vi "Test_HW_Stream_raw_data_channel.vi"(7 "At least bits":u32=30, 8 "error in":errorcluster, 9 "Event Type":T1=1073684533 items=["Service Request"=1073684491, "Trigger"=3221168138, "Clear"=1073684493, "VXI Signal"=1073684512, "VXI/VME Interrupt"=3221168161, "VXI/VME Sysfail"=1073684509, "VXI/VME Sysreset"=1073684510, "GPIB CIC"=1073684498, "GPIB Talk"=1073684499, "GPIB Listen"=1073684500, "PXI Interrupt"=1073684514, "Serial Break"=1073684515, "Serial TermChar"=1073684516, "Serial CTS"=1073684521, "Serial DSR"=1073684522, "Serial DCD"=1073684524, "Serial RI"=1073684526, "Serial Character"=1073684533, "USB Interrupt"=1073684535, "All Enabled"=1073709055], 10 "Data flow controls in":T3, 11 "VISA resource name in":refnum<visa-resource-name>) -> (0 "error out":errorcluster, 1 "High-speed channel":T2, 2 "Data flow controls out":T3, 3 "VISA resource name out":refnum<visa-resource-name>, 4 "Timestamp":timestamp, 6 "Time to process, us":dbl format="%0.2f")   [LabVIEW 2018]
uses:
  <extravilib>/ChannelInstances/High Speed Stream-c(a[.](u16),stamp,str)/)Channel.ctl
  <vilib>/Instr/_visa.llb/Select Event Type.ctl
  <vilib>/Instr/_visa.llb/VISA Flush IO Buffer Mask.ctl
  <extravilib>/ChannelInstances/High Speed Stream-c(a[.](u16),stamp,str).lvlib
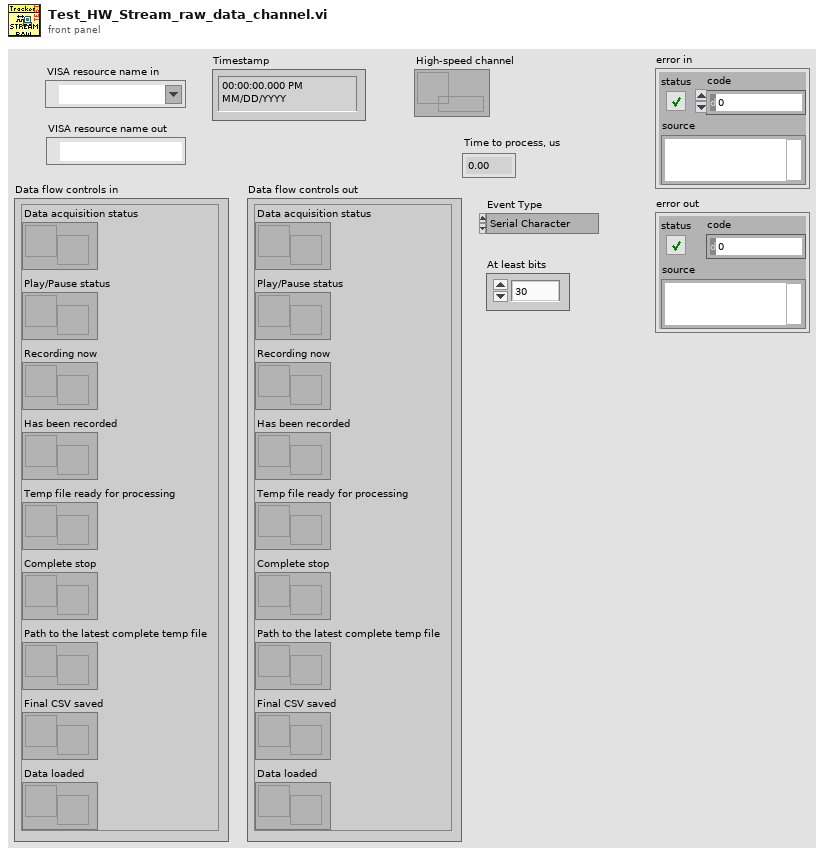
[diagram p1: front panel]
types:
  T1 = typedef "Select Event Type.ctl" = u32
  T2 = typedef "High Speed Stream-c(a[.](u16),stamp,str).lvlib/)Channel.ctl" = refnum<queue>
  T3 = cluster{"Data acquisition status":refnum<notifier>, "Play/Pause status":refnum<notifier>, "Complete stop":refnum<notifier>, "Temp file ready for processing":refnum<notifier>, "Has been recorded":refnum<notifier>, "Recording now":refnum<notifier>, "Path to the latest complete temp file":refnum<notifier>, "Final CSV saved":refnum<notifier>, "Data loaded":refnum<notifier>}
  T4 = typedef "VISA Flush IO Buffer Mask.ctl" = u16
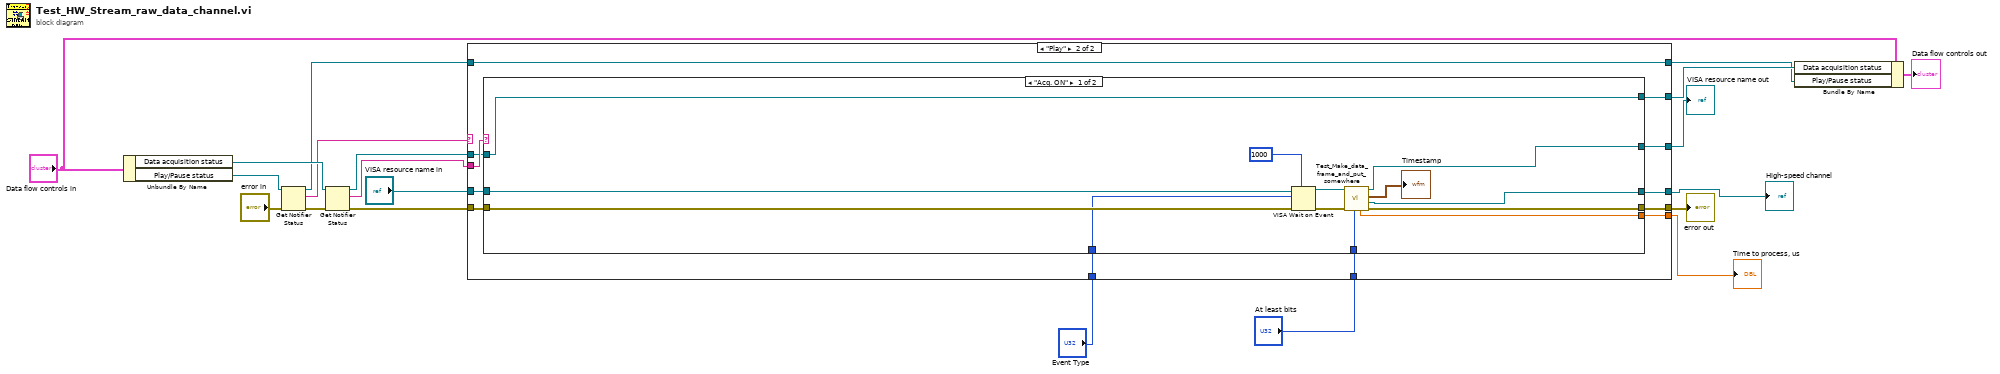
[diagram p0: block diagram]
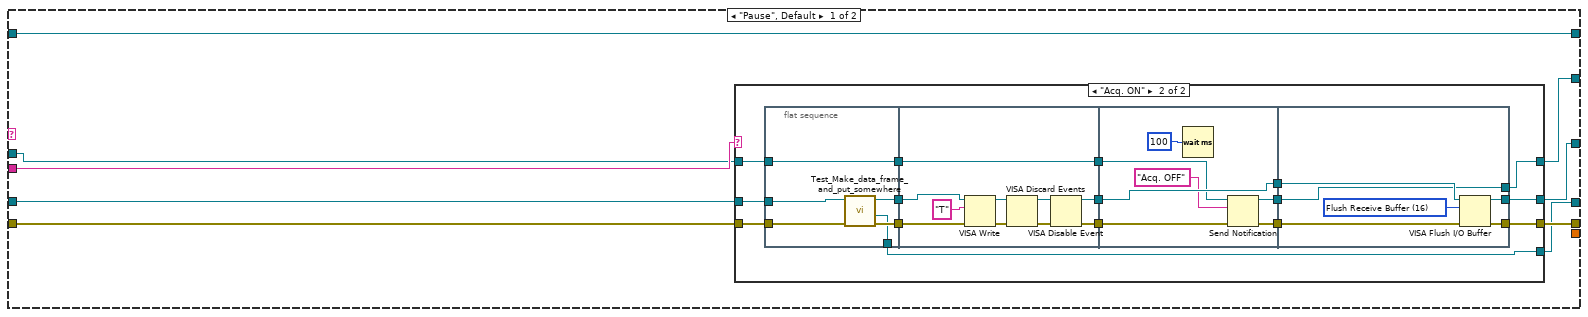
[diagram p2: hidden frame]
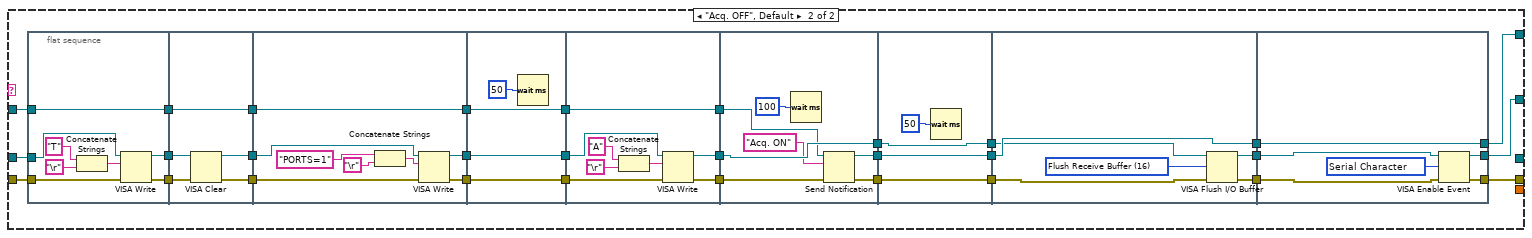
[diagram p4: hidden frame]
diagram:
  n1 = Unbundle By Name("Data flow controls in") -> ("Data acquisition status"=w18:refnum<notifier>, "Play/Pause status"=w17:refnum<notifier>)
  n2 = Get Notifier Status(notifier=w17, error in (no error)="error in") -> (notifier out=w12:refnum<notifier>, current notification=w16:string, error out=w13:errorcluster)  [unwired: 2 out]
  n3 = Get Notifier Status(notifier=w18, error in (no error)=w13) -> (notifier out=w11:refnum<notifier>, current notification=w15:string, error out=w6:errorcluster)  [unwired: 2 out]
  n4 = case shown="\"Play\"" w16 {
    tunnel: [w24 w84] -> w19
    tunnel: "VISA resource name in" -> [w29 w89]
    tunnel: w15 -> [w28 w87]
    tunnel: w12 -> [w26 w85]
    tunnel: w11 -> [w27 w86]
    tunnel: [w23 w83] -> w9
    tunnel: [w26 w85] -> w8
    tunnel: w6 -> [w25 w88]
    tunnel: [w22 w82] -> w5
    tunnel: [_ w81] -> w4
    tunnel: [w21 w80] -> w1
    tunnel: "Event Type" -> [_ w79]
    tunnel: "At least bits" -> [_ w78]
    frame "Pause", Default {
      n5 = case shown="\"Acq. ON\"" w28 {
        tunnel: w29 -> [w32 w46]
        tunnel: [w32 w45] -> w24
        tunnel: w27 -> [w31 w39]
        tunnel: [w31 w38] -> w23
        tunnel: w25 -> [w30 w42]
        tunnel: [w30 w41] -> w22
        tunnel: [_ w33] -> w21
        frame "Acq. OFF", Default {
        }
        frame "Acq. ON" {
          n6 = flat-sequence {
            tunnel: w39 -> [w54]
            tunnel: w42 -> [w53]
            tunnel: w46 -> [w51]
            tunnel: [w50] -> w36
            tunnel: [w52] -> w35
            tunnel: [w54] -> w34
            tunnel: [w49] -> w33
            tunnel: [w56] -> w48
            tunnel: [w55] -> w47
            tunnel: [w64] -> w40
            tunnel: w36 -> [w62]
            tunnel: w35 -> [w61]
            tunnel: w34 -> [w64]
            tunnel: w48 -> [w70]
            tunnel: w47 -> [w69]
            tunnel: [w70] -> w44
            tunnel: [w68] -> w43
            tunnel: w40 -> [w66]
            tunnel: [w65] -> w37
            tunnel: [w75] -> w45
            tunnel: w44 -> [w76]
            tunnel: w43 -> [w77]
            tunnel: [w73] -> w41
            tunnel: [w72] -> w38
            tunnel: w37 -> [w72]
            frame #0 {
              n7 = call "Test_Make_data_frame_and_put_somewhere.vi"("error in"=w53, "VISA resource name in"=w51) -> ("error out"=w52:errorcluster, "High-speed channel"=w49:T2, "VISA resource name out"=w50:refnum<visa-resource-name>)  [unwired: 5 in, 2 out]
            }
            frame #1 {
              n8 = VISA Write(VISA resource name=w62, write buffer="T", error in (no error)=w61) -> (VISA resource name out=w59:refnum<visa-resource-name>, error out=w60:errorcluster)  [unwired: 1 out]
              n9 = VISA Discard Events(8:w60, 11:w59) -> (0:w58:errorcluster, 3:w57:refnum<visa-resource-name>)  [unwired: 2 in]
              n10 = VISA Disable Event(8:w58, 11:w57) -> (0:w55:errorcluster, 3:w56:refnum<visa-resource-name>)  [unwired: 2 in]
            }
            frame #2 {
              n11 = Wait (ms)(milliseconds to wait=u32 100) -> ()  [unwired: 1 out]
              n12 = Send Notification(notification="Acq. OFF", notifier=w66, error in (no error)=w69) -> (notifier out=w65:refnum<notifier>, error out=w68:errorcluster)
            }
            frame #3 {
              w74 = T4 16 items=["Flush Receive Buffer"=16, "Write Transmit Buffer to Device"=32, "Flush Receive Buffer (No I/O)"=64, "Flush Transmit Buffer"=128] ("Mask")
              n13 = VISA Flush I/O Buffer(VISA resource name=w76, mask (16)=w74, error in (no error)=w77) -> (VISA resource name out=w75:refnum<visa-resource-name>, error out=w73:errorcluster)
            }
          }
        }
      }
    }
    frame "Play" {
      n14 = case shown="\"Acq. ON\"" w87 {
        tunnel: w89 -> [w96 w130]
        tunnel: [w99 w103] -> w84
        tunnel: [w100 w104] -> w82
        tunnel: w88 -> [w98 w123]
        tunnel: w86 -> [w102 w118]
        tunnel: [w102 w117] -> w83
        tunnel: [w93 _] -> w81
        tunnel: [w92 _] -> w80
        tunnel: w79 -> [w91 _]
        tunnel: w78 -> [w90 _]
        frame "Acq. ON" {
          n15 = VISA Wait on Event(7:u32 1000 ("timeout (0)"), 8:w98, 10:w91, 11:w96) -> (0:w97:errorcluster, 3:w95:refnum<visa-resource-name>)  [unwired: 1 in, 2 out]
          n16 = call "Test_Make_data_frame_and_put_somewhere.vi"("At least bits"=w90, "error in"=w97, "VISA resource name in"=w95) -> ("error out"=w100:errorcluster, "High-speed channel"=w92:T2, "Timestamp"=→"Timestamp":timestamp, "VISA resource name out"=w99:refnum<visa-resource-name>, "Time to process, us"=w93:dbl)  [unwired: 4 in]
        }
        frame "Acq. OFF", Default {
          n17 = flat-sequence {
            tunnel: w130 -> [w139]
            tunnel: [w140] -> w129
            tunnel: [w138] -> w128
            tunnel: w123 -> [w134]
            tunnel: [w133] -> w119
            tunnel: w118 -> [w133]
            tunnel: [w145] -> w125
            tunnel: [w144] -> w124
            tunnel: w128 -> [w143]
            tunnel: w129 -> [w142]
            tunnel: [w141] -> w120
            tunnel: w119 -> [w141]
            tunnel: w125 -> [w151]
            tunnel: [w150] -> w127
            tunnel: w124 -> [w149]
            tunnel: [w148] -> w126
            tunnel: [w146] -> w121
            tunnel: w120 -> [w146]
            tunnel: [w156] -> w110
            tunnel: [w155] -> w109
            tunnel: [w157] -> w108
            tunnel: w121 -> [w157]
            tunnel: w127 -> [w156]
            tunnel: w126 -> [w155]
            tunnel: [w160] -> w132
            tunnel: [w159] -> w131
            tunnel: w110 -> [w162]
            tunnel: w109 -> [w161]
            tunnel: [w158] -> w122
            tunnel: w108 -> [w158]
            tunnel: w132 -> [w170]
            tunnel: w131 -> [w171]
            tunnel: w122 -> [w168]
            tunnel: [w169] -> w116
            tunnel: [w171] -> w115
            tunnel: [w167] -> w114
            tunnel: w116 -> [w176]
            tunnel: [w176] -> w113
            tunnel: w115 -> [w175]
            tunnel: [w175] -> w112
            tunnel: w114 -> [w174]
            tunnel: [w174] -> w111
            tunnel: w111 -> [w178]
            tunnel: w112 -> [w177]
            tunnel: w113 -> [w179]
            tunnel: [w181] -> w107
            tunnel: [w182] -> w106
            tunnel: [w178] -> w105
            tunnel: [w188] -> w117
            tunnel: w107 -> [w186]
            tunnel: w106 -> [w185]
            tunnel: w105 -> [w188]
            tunnel: [w187] -> w104
            tunnel: [w184] -> w103
            frame #0 {
              n18 = Concatenate Strings("T" ("write buffer"), "\r") -> (w135:string)
              n19 = VISA Write(VISA resource name=w139, write buffer=w135, error in (no error)=w134) -> (VISA resource name out=w140:refnum<visa-resource-name>, error out=w138:errorcluster)  [unwired: 1 out]
            }
            frame #1 {
              n20 = VISA Clear(VISA resource name=w142, error in (no error)=w143) -> (VISA resource name out=w145:refnum<visa-resource-name>, error out=w144:errorcluster)
            }
            frame #2 {
              n21 = Concatenate Strings("PORTS=1" ("write buffer"), "\r") -> (w152:string)
              n22 = VISA Write(VISA resource name=w151, write buffer=w152, error in (no error)=w149) -> (VISA resource name out=w150:refnum<visa-resource-name>, error out=w148:errorcluster)  [unwired: 1 out]
            }
            frame #3 {
              n23 = Wait (ms)(milliseconds to wait=u32 50) -> ()  [unwired: 1 out]
            }
            frame #4 {
              n24 = Concatenate Strings("A" ("write buffer"), "\r") -> (w163:string)
              n25 = VISA Write(VISA resource name=w162, write buffer=w163, error in (no error)=w161) -> (VISA resource name out=w159:refnum<visa-resource-name>, error out=w160:errorcluster)  [unwired: 1 out]
            }
            frame #5 {
              n26 = Wait (ms)(milliseconds to wait=u32 100) -> ()  [unwired: 1 out]
              n27 = Send Notification(notification="Acq. ON", notifier=w168, error in (no error)=w170) -> (notifier out=w167:refnum<notifier>, error out=w169:errorcluster)
            }
            frame #6 {
              n28 = Wait (ms)(milliseconds to wait=u32 50) -> ()  [unwired: 1 out]
            }
            frame #7 {
              w180 = T4 16 items=["Flush Receive Buffer"=16, "Write Transmit Buffer to Device"=32, "Flush Receive Buffer (No I/O)"=64, "Flush Transmit Buffer"=128] ("Mask")
              n29 = VISA Flush I/O Buffer(VISA resource name=w177, mask (16)=w180, error in (no error)=w179) -> (VISA resource name out=w182:refnum<visa-resource-name>, error out=w181:errorcluster)
            }
            frame #8 {
              w183 = T1 1073684533 items=["Service Request"=1073684491, "Trigger"=3221168138, "Clear"=1073684493, "VXI Signal"=1073684512, "VXI/VME Interrupt"=3221168161, "VXI/VME Sysfail"=1073684509, "VXI/VME Sysreset"=1073684510, "GPIB CIC"=1073684498, "GPIB Talk"=1073684499, "GPIB Listen"=1073684500, "PXI Interrupt"=1073684514, "Serial Break"=1073684515, "Serial TermChar"=1073684516, "Serial CTS"=1073684521, "Serial DSR"=1073684522, "Serial DCD"=1073684524, "Serial RI"=1073684526, "Serial Character"=1073684533, "USB Interrupt"=1073684535, "All Enabled"=1073709055] ("Event Type")
              n30 = VISA Enable Event(8:w186, 10:w183, 11:w185) -> (0:w187:errorcluster, 3:w184:refnum<visa-resource-name>)  [unwired: 1 in]
            }
          }
        }
      }
    }
  }
  "VISA resource name out" <- w19
  "error out" <- w5
  "Time to process, us" <- w4
  "High-speed channel" <- w1
  n31 = Bundle By Name(cluster="Data flow controls in", "Data acquisition status"=w9, "Play/Pause status"=w8) -> (→"Data flow controls out":T3)
